vi "Type.vi"(11 "json class in":refnum<class "json class.lvclass">) -> (2 "Name":string)   [LabVIEW 2025, in "Config Library.lvlib" / "json class.lvclass"]
uses:
  json class.lvclass
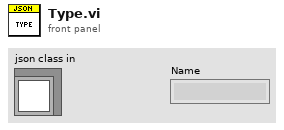
[diagram p1: front panel]
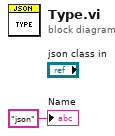
[diagram p0: block diagram]
diagram:
  "Name" <- "json" ("Name")
